vi "Perform Action.vi"(8 "error in":errorcluster, 10 "Input":variant, 11 "DO DAQmx Fixed Freq PWM CFG in":refnum<class "DO DAQmx Fixed Freq PWM CFG.lvclass">) -> (0 "error out":errorcluster, 2 "Output":variant, 3 "DO DAQmx Fixed Freq PWM CFG out":refnum<class "DO DAQmx Fixed Freq PWM CFG.lvclass">)   [LabVIEW 2024, in "DO DAQmx Fixed Freq PWM CFG.lvclass"]
uses:
  DO DAQmx Fixed Freq PWM CFG.lvclass
  DAQmx Base CFG/DAQmx Base CFG.lvclass/DAQmx Base CFG.ctl
  DO DAQmx Fixed Freq PWM CFG.lvclass/DO DAQmx Fixed Freq PWM CFG.ctl
  <vilib>/DAQmx/write.llb/DAQmx Write (Digital 1D Wfm NChan NSamp).vi
  <vilib>/Waveform/DWDTOps.llb/DWDT Uncompress Digital.vi
  <vilib>/DAQmx/miscellaneous.llb/DAQmx Fill In Error Info.vi
  DAQmx Base CFG/DAQmx Base CFG.lvclass
  D:/git/HAL/HAL/Devices/DAQmx/DAQmx Base CFG/DAQmx Base CFG.lvclass
  D:/git/HAL/HAL/Configurations/CFG JSON/CFG JSON.lvclass
  D:/git/HAL/HAL/Configurations/CFG Base/CFG Base.lvclass
  D:/git/HAL/HAL/Devices/DAQmx/DIO/DO DAQmx Fixed Freq PWM CFG/DO DAQmx Fixed Freq PWM CFG.lvclass
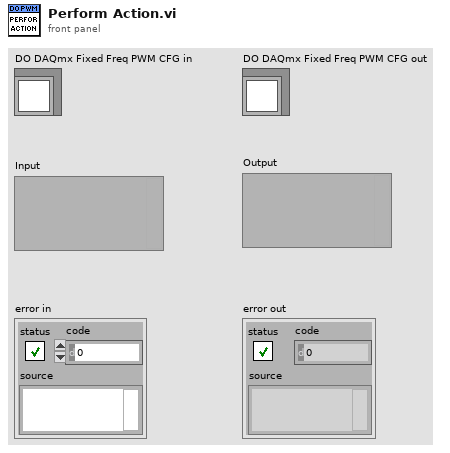
[diagram p1: front panel]
types:
  T1 = cluster{"Samplerate":dbl, "Samples per Channel":u32}
  T2 = cluster{"Channel":string, "Digital Waveform":digitalwaveform}[]
  T3 = cluster{"Channel":string, "digital waveform":digitalwaveform}
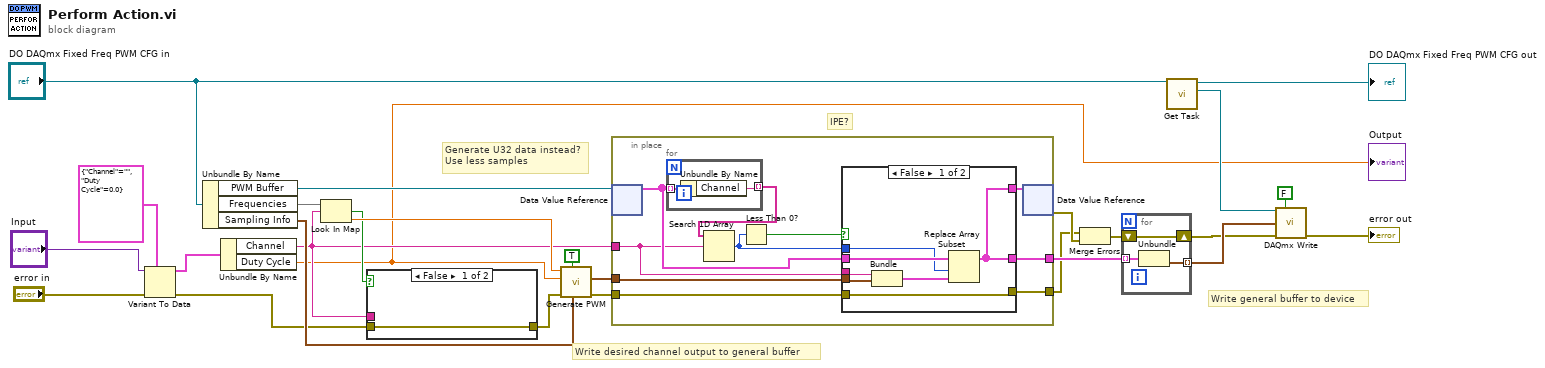
[diagram p0: block diagram]
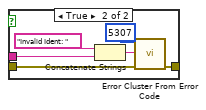
[diagram p2: hidden frame]
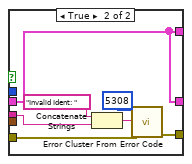
[diagram p3: hidden frame]
diagram:
  # "Generate U32 data instead?\nUse less samples"
  # "IPE?"
  # "Write general buffer to device"
  # "Write desired channel output to general buffer"
  n1 = Variant To Data(error in="error in", type=cluster{"Channel":string, "Duty Cycle":dbl} {"Channel"="", "Duty Cycle"=0.0}, Variant="Input") -> (data=w27:cluster{"Channel":string, "Duty Cycle":dbl}, error out=w12:errorcluster)
  n2 = Unbundle By Name("DO DAQmx Fixed Freq PWM CFG in") -> ("PWM Buffer"=w24:refnum<data-value>, "Frequencies"=w14:map{string, dbl}, "Sampling Info"=w15:T1)
  n3 = Unbundle By Name(w27) -> ("Channel"=w9:string, "Duty Cycle"=w2:dbl)
  "Output" <- w2
  n4 = Look In Map(map=w14, key=w9) -> (key not found?=w11:bool, value=w13:dbl)  [unwired: 1 in]
  n5 = case shown="False" w11 {
    tunnel: w12 -> [w28 w29]
    tunnel: [w28 w34] -> w10
    tunnel: w9 -> [_ w31]
    frame False {
    }
    frame True {
      n6 = Concatenate Strings("Invalid Ident: ", w31) -> (w33:string)
      n7 = call <vilib>:"Error Cluster From Error Code.vi"("error in (no error)"=w29, "error message (\"\")"=w33, "error code (0)"=5307) -> ("error out"=w34:errorcluster)  [unwired: 6 in]
    }
  }
  n8 = call "Generate PWM.vi"("sampling info"=w15, "reset?"=TRUE, "error in"=w10, "duty cycle"=w2, "frequency"=w13) -> ("error out"=w8:errorcluster, "digital waveform"=w23:digitalwaveform)  [unwired: 5 in]
  n9 = in-place {
    in-place-border: w9 -> [w38]
    in-place-border: w23 -> [w37]
    in-place-border: [w35] -> w21
    in-place-border: w8 -> [w41]
    in-place-border: [w40] -> w7
    n10 = in-place-dvr #1(w24) -> (w39:T2)  [unwired: 1 out]
    n11 = for {
      tunnel: w39 -> [w60] mode=indexing
      tunnel: [w59] -> w44 mode=indexing
      n12 = Unbundle By Name(w60) -> ("Channel"=w59:string)
    }
    n13 = Search 1D Array(1D array=w44, element=w38) -> (index of element=w42:i32)  [unwired: 1 in]
    n14 = Less Than 0?(x=w42) -> (x < 0?=w43:bool)
    n15 = case shown="False" w43 {
      tunnel: w42 -> [w49 _]
      tunnel: w41 -> [w51 w55]
      tunnel: [w51 w54] -> w40
      tunnel: w39 -> [w50 w52]
      tunnel: w38 -> [w48 w53]
      tunnel: w37 -> [w47 _]
      tunnel: [w45 w52] -> w36
      tunnel: [w45 w52] -> w35
      frame False {
        n16 = Bundle("Channel"=w48, "digital waveform"=w47) -> (w46:T3)  [unwired: 1 in]
        n17 = Replace Array Subset(array=w50, new element=w46, index=w49) -> (w45:T2)
      }
      frame True {
        n18 = Concatenate Strings("Invalid Ident: ", w53) -> (w58:string)
        n19 = call <vilib>:"Error Cluster From Error Code.vi"("error in (no error)"=w55, "error message (\"\")"=w58, "error code (0)"=5308) -> ("error out"=w54:errorcluster)  [unwired: 6 in]
      }
    }
    n20 = in-place-dvr #1(w36) -> (w19:errorcluster)  [unwired: 1 out]
  }
  n21 = Merge Errors(w7, w19) -> (w18:errorcluster)
  n22 = for {
    tunnel: w21 -> [w63] mode=indexing
    tunnel: [w62] -> w20 mode=indexing
    shift-right: [w61] -> w5
    shift-left: w18 -> [w61]
    n23 = Unbundle(w63) -> ("Digital Waveform"=w62:digitalwaveform)  [unwired: 1 out]
  }
  n24 = call "Get Task.vi"("DAQmx Base CFG in"="DO DAQmx Fixed Freq PWM CFG in") -> ("Task"=w22:refnum<k21>, "DAQmx Base CFG out"=→"DO DAQmx Fixed Freq PWM CFG out":refnum<class "DO DAQmx Fixed Freq PWM CFG.lvclass">)  [unwired: 9 in]
  n25 = call-poly <vilib>:"DAQmx Write.vi"("task/channels in"=w22, "auto start"=FALSE, "data"=w20, "error in"=w5) -> ("error out"=→"error out":errorcluster)  [unwired: 9 in, 2 out]
